vi "Alarm_CompareToThresholds.vi"(11 "HDF5_file_refs":T4 {"10HzRefs"."FileRef" format="%.0x"; "10HzRefs"."84Co_dset" format="%.0x"; "10HzRefs"."72Co_dset" format="%.0x"; "AlarmCfg"."84X_CalTonePwr"."ErrsAndWarns" scale=-120.0..-45.0; "AlarmCfg"."72X_CalTonePwr"."ErrsAndWarns" scale=-120.0..-45.0; "AlarmCfg"."84Co_CalTonePwr"."ErrsAndWarns" scale=-120.0..-45.0; "AlarmCfg"."72Co_CalTonePwr"."ErrsAndWarns" scale=-120.0..-45.0; "AlarmCfg"."84CoCalFreq"."ErrsAndWarns" scale=24.9..25.1; "AlarmCfg"."84CoBeacFreq"."ErrsAndWarns" scale=25.5..27.0; "AlarmCfg"."72CoCalFreq"."ErrsAndWarns" scale=24.9..25.1; "AlarmCfg"."72CoBeacFreq"."ErrsAndWarns" scale=25.5..27.0; "AlarmCfg"."ADAM4"."ErrsAndWarns" scale=30.0..52.0; "AlarmCfg"."ADAM3"."ErrsAndWarns" scale=30.0..52.0; "AlarmCfg"."ADAM2"."ErrsAndWarns" scale=30.0..52.0; "AlarmCfg"."ADAM1"."ErrsAndWarns" scale=30.0..52.0; "AlarmCfg"."TE3"."ErrsAndWarns" scale=30.0..52.0; "AlarmCfg"."TE2"."ErrsAndWarns" scale=30.0..52.0; "AlarmCfg"."TE1"."ErrsAndWarns" scale=20.0..52.0; "AlarmCfg"."AI19"."ErrsAndWarns" scale=0.0..60.0; "AlarmCfg"."AI18"."ErrsAndWarns" scale=-10.0..10.0; "AlarmCfg"."AI6"."ErrsAndWarns" scale=0.0..35.0; "AlarmCfg"."AI5"."ErrsAndWarns" scale=0.0..20.0; "AlarmCfg"."AI4"."ErrsAndWarns" scale=0.0..15.0; "AlarmCfg"."AI3"."ErrsAndWarns" scale=0.0..10.0; "AlarmCfg"."AI2"."ErrsAndWarns" scale=0.0..10.0; "AlarmCfg"."TC13"."ErrsAndWarns" scale=-10.0..40.0; "LogData"."NoiseInfo"."HDF5_NoiseInfo"."Sum" format="%^#.1g"; "HDFRefs2"."Complex"."Group_ref" format="%.0x"; "HDFRefs2"."Complex"."QSpect_dset" format="%.0x"; "HDFRefs2"."Complex"."ISpect_dset" format="%.0x"; "HDFRefs2"."Complex"."PwrSpect_dset" format="%.0x"; "HDFRefs2"."Complex"."TImeStamp_dset" format="%.0x"; "HDFRefs2"."ADAM_Refs"."Group_ref" format="%.0x"; "HDFRefs2"."ADAM_Refs"."ADAM_CoPol_dset" format="%.0x"; "HDFRefs2"."ADAM_Refs"."ADAM_XPol_dset" format="%.0x"; "HDFRefs2"."ADAM_Refs"."ADAM_Noise_dset" format="%.0x"; "HDFRefs2"."ADAM_Refs"."ADAM_CalBox_dset" format="%.0x"; "HDFRefs2"."ADAM_Refs"."TimeStamp" format="%.0x"; "HDFRefs2"."Filter_Refs"."Filter_Group_ref" format="%.0x"; "HDFRefs2"."Filter_Refs"."TimeStamp_dset" format="%.0x"; "HDFRefs2"."Filter_Refs"."Filter_dset" format="%.0x"; "HDFRefs2"."AI_Refs"."BlowerPwr_dset" format="%.0x"; "HDFRefs2"."AI_Refs"."ElStdDev_dset" format="%.0x"; "HDFRefs2"."AI_Refs"."AzStdDev_dset" format="%.0x"; "HDFRefs2"."AI_Refs"."AI19_dset" format="%.0x"; "HDFRefs2"."AI_Refs"."AI18_dset" format="%.0x"; "HDFRefs2"."AI_Refs"."AI17_dset" format="%.0x"; "HDFRefs2"."AI_Refs"."AI16_dset" format="%.0x"; "HDFRefs2"."AI_Refs"."AI6_dset" format="%.0x"; "HDFRefs2"."AI_Refs"."AI5_dset" format="%.0x"; "HDFRefs2"."AI_Refs"."AI4_dset" format="%.0x"; "HDFRefs2"."AI_Refs"."AI3_dset" format="%.0x"; "HDFRefs2"."AI_Refs"."AI2_dset" format="%.0x"; "HDFRefs2"."AI_Refs"."AI0_dset" format="%.0x"; "HDFRefs2"."AI_Refs"."AI1_dset" format="%.0x"; "HDFRefs2"."AI_Refs"."TimeString_dset" format="%.0x"; "HDFRefs2"."AI_Refs"."TimeStamp_dset" format="%.0x"; "HDFRefs2"."AI_Refs"."Group_ref" format="%.0x"; "HDFRefs2"."Weath_Refs"."WindDirSTD_dset" format="%.0x"; "HDFRefs2"."Weath_Refs"."WindGusts_dset" format="%.0x"; "HDFRefs2"."Weath_Refs"."RainFall_dset" format="%.0x"; "HDFRefs2"."Weath_Refs"."RainRate_dset" format="%.0x"; "HDFRefs2"."Weath_Refs"."Pressure_dset" format="%.0x"; "HDFRefs2"."Weath_Refs"."Humidity_dset" format="%.0x"; "HDFRefs2"."Weath_Refs"."Temp_dset" format="%.0x"; "HDFRefs2"."Weath_Refs"."WindDir_dset" format="%.0x"; "HDFRefs2"."Weath_Refs"."WindSpd_dset" format="%.0x"; "HDFRefs2"."Weath_Refs"."TimeStamp_dset" format="%.0x"; "HDFRefs2"."Weath_Refs"."Group_ref" format="%.0x"; "HDFRefs2"."Weath_Refs"."TimeString_dset" format="%.0x"; "HDFRefs2"."UPS_Refs_Deprecated"."TimeStamp_dset" format="%.0x"; "HDFRefs2"."UPS_Refs_Deprecated"."TimeString_dset" format="%.0x"; "HDFRefs2"."UPS_Refs_Deprecated"."%_dset" format="%.0x"; "HDFRefs2"."UPS_Refs_Deprecated"."W_dset" format="%.0x"; "HDFRefs2"."UPS_Refs_Deprecated"."Hz_dset" format="%.0x"; "HDFRefs2"."UPS_Refs_Deprecated"."A_dset" format="%.0x"; "HDFRefs2"."UPS_Refs_Deprecated"."V_dset" format="%.0x"; "HDFRefs2"."UPS_Refs_Deprecated"."Group_ref" format="%.0x"; "HDFRefs2"."TE_Refs"."TimeStamp" format="%.0x"; "HDFRefs2"."TE_Refs"."TE_Outp3_dset" format="%.0x"; "HDFRefs2"."TE_Refs"."TE_Temp3_dset" format="%.0x"; "HDFRefs2"."TE_Refs"."TE_Outp2_dset" format="%.0x"; "HDFRefs2"."TE_Refs"."TE_Temp2_dset" format="%.0x"; "HDFRefs2"."TE_Refs"."TE_Outp1_dset" format="%.0x"; "HDFRefs2"."TE_Refs"."TE_Temp1_dset" format="%.0x"; "HDFRefs2"."TE_Refs"."Group_ref" format="%.0x"; "HDFRefs2"."DisdromRefs"."Status_dset_deprecated" format="%.0x"; "HDFRefs2"."DisdromRefs"."Spectrum_dset" format="%.0x"; "HDFRefs2"."DisdromRefs"."SpectGroup_ref" format="%.0x"; "HDFRefs2"."DisdromRefs"."HydromType_dset" format="%.0x"; "HDFRefs2"."DisdromRefs"."UnknownVolum_dset" format="%.0x"; "HDFRefs2"."DisdromRefs"."UnknownParticls_dset" format="%.0x"; "HDFRefs2"."DisdromRefs"."NonHydrVolum_dset" format="%.0x"; "HDFRefs2"."DisdromRefs"."NonHydrParticls_dset" format="%.0x"; "HDFRefs2"."DisdromRefs"."ParticlMinDiam_dset" format="%.0x"; "HDFRefs2"."DisdromRefs"."ParticlMaxSpeed_dset" format="%.0x"; "HDFRefs2"."DisdromRefs"."RadarReflect_dset" format="%.0x"; "HDFRefs2"."DisdromRefs"."Visibility_dset" format="%.0x"; "HDFRefs2"."DisdromRefs"."TotalRain_dset" format="%.0x"; "HDFRefs2"."DisdromRefs"."Solid_dset" format="%.0x"; "HDFRefs2"."DisdromRefs"."Liquid_dset" format="%.0x"; "HDFRefs2"."DisdromRefs"."TotalRainRate_dset" format="%.0x"; "HDFRefs2"."DisdromRefs"."TimeStamp_dset" format="%.0x"; "HDFRefs2"."DisdromRefs"."ParticlMinSpeed_dset" format="%.0x"; "HDFRefs2"."DisdromRefs"."MeasdParticles_dset" format="%.0x"; "HDFRefs2"."DisdromRefs"."MaxDiam_dset" format="%.0x"; "HDFRefs2"."DisdromRefs"."BasicGroup_ref" format="%.0x"; "HDFRefs2"."ValidRefs"."Alarm_Source_dset" format="%.0x"; "HDFRefs2"."ValidRefs"."Time_AlarmChange_dset" format="%.0x"; "HDFRefs2"."ValidRefs"."Time_Valid_dset" format="%.0x"; "HDFRefs2"."ValidRefs"."Alarm_Valid_dset" format="%.0x"; "HDFRefs2"."ValidRefs"."Saturat_dset" format="%.0x"; "HDFRefs2"."ValidRefs"."Group_ref" format="%.0x"; "HDFRefs2"."ValidRefs"."Weath_Valid_dset" format="%.0x"; "HDFRefs2"."ValidRefs"."Disdr_Valid_dset" format="%.0x"; "HDFRefs2"."TC_Refs"."TC13_Tamb_Inter" format="%.0x"; "HDFRefs2"."TC_Refs"."TC12_Gen_Exhaust" format="%.0x"; "HDFRefs2"."TC_Refs"."TC11_HVAC_Cond_Out" format="%.0x"; "HDFRefs2"."TC_Refs"."TC10_HVAC_Cond_In" format="%.0x"; "HDFRefs2"."TC_Refs"."TC9_LP2_Lo" format="%.0x"; "HDFRefs2"."TC_Refs"."TC8_LP2_LoMid" format="%.0x"; "HDFRefs2"."TC_Refs"."TC7_LP2_Mid" format="%.0x"; "HDFRefs2"."TC_Refs"."TC6_LP2_MidHi" format="%.0x"; "HDFRefs2"."TC_Refs"."TC5_LP2_Hi" format="%.0x"; "HDFRefs2"."TC_Refs"."TC4_LP1_Lo" format="%.0x"; "HDFRefs2"."TC_Refs"."TC3_LP1_LoMid" format="%.0x"; "HDFRefs2"."TC_Refs"."TC2_LP1_Mid" format="%.0x"; "HDFRefs2"."TC_Refs"."TC1_LP1_MidHi" format="%.0x"; "HDFRefs2"."TC_Refs"."TC0_LP1_Hi" format="%.0x"; "HDFRefs2"."TC_Refs"."TimeString_dset" format="%.0x"; "HDFRefs2"."TC_Refs"."TimeStamp_dset" format="%.0x"; "HDFRefs2"."TC_Refs"."Group_ref" format="%.0x"; "HDFRefs2"."NoiseRefs"."TimeStamp_df_dset" format="%.0x"; "HDFRefs2"."NoiseRefs"."sum_dset" format="%.0x"; "HDFRefs2"."NoiseRefs"."df_dset" format="%.0x"; "HDFRefs2"."NoiseRefs"."TimeStamp_dset" format="%.0x"; "HDFRefs2"."NoiseRefs"."SumdSpectrum_dset" format="%.0x"; "HDFRefs2"."NoiseRefs"."TimeString_dset" format="%.0x"; "HDFRefs2"."NoiseRefs"."Group_ref" format="%.0x"; "HDFRefs2"."ToneRefs"."Group_ref" format="%.0x"; "HDFRefs2"."ToneRefs"."Cal"."Downshift_dset" format="%.0x"; "HDFRefs2"."ToneRefs"."Cal"."DeltaPhase_dset" format="%.0x"; "HDFRefs2"."ToneRefs"."Cal"."Phase_dset" format="%.0x"; "HDFRefs2"."ToneRefs"."Cal"."SNR_dset" format="%.0x"; "HDFRefs2"."ToneRefs"."Cal"."df_dset" format="%.0x"; "HDFRefs2"."ToneRefs"."Cal"."PeakLoc_dset" format="%.0x"; "HDFRefs2"."ToneRefs"."Cal"."MaxValue_dset" format="%.0x"; "HDFRefs2"."ToneRefs"."Cal"."TImeStamp_dset" format="%.0x"; "HDFRefs2"."ToneRefs"."Cal"."TimeString_dset" format="%.0x"; "HDFRefs2"."ToneRefs"."Beac"."Downshift_dset" format="%.0x"; "HDFRefs2"."ToneRefs"."Beac"."DeltaPhase_dset" format="%.0x"; "HDFRefs2"."ToneRefs"."Beac"."Phase_dset" format="%.0x"; "HDFRefs2"."ToneRefs"."Beac"."SNR_dset" format="%.0x"; "HDFRefs2"."ToneRefs"."Beac"."df_dset" format="%.0x"; "HDFRefs2"."ToneRefs"."Beac"."PeakLoc_dset" format="%.0x"; "HDFRefs2"."ToneRefs"."Beac"."MaxValue_dset" format="%.0x"; "HDFRefs2"."ToneRefs"."Beac"."TImeStamp_dset" format="%.0x"; "HDFRefs2"."ToneRefs"."Beac"."TimeString_dset" format="%.0x"; "HDFRefs2"."ToneRefs"."CalZoom_dSet" format="%.0x"; "HDFRefs2"."ToneRefs"."BeacZoom_dSet" format="%.0x"; "HDFRefs2"."File" format="%.0x"; "HDFRefs1"."Complex"."Group_ref" format="%.0x"; "HDFRefs1"."Complex"."QSpect_dset" format="%.0x"; "HDFRefs1"."Complex"."ISpect_dset" format="%.0x"; "HDFRefs1"."Complex"."PwrSpect_dset" format="%.0x"; "HDFRefs1"."Complex"."TImeStamp_dset" format="%.0x"; "HDFRefs1"."ADAM_Refs"."Group_ref" format="%.0x"; "HDFRefs1"."ADAM_Refs"."ADAM_CoPol_dset" format="%.0x"; "HDFRefs1"."ADAM_Refs"."ADAM_XPol_dset" format="%.0x"; "HDFRefs1"."ADAM_Refs"."ADAM_Noise_dset" format="%.0x"; "HDFRefs1"."ADAM_Refs"."ADAM_CalBox_dset" format="%.0x"; "HDFRefs1"."ADAM_Refs"."TimeStamp" format="%.0x"; "HDFRefs1"."Filter_Refs"."Filter_Group_ref" format="%.0x"; "HDFRefs1"."Filter_Refs"."TimeStamp_dset" format="%.0x"; "HDFRefs1"."Filter_Refs"."Filter_dset" format="%.0x"; "HDFRefs1"."AI_Refs"."BlowerPwr_dset" format="%.0x"; "HDFRefs1"."AI_Refs"."ElStdDev_dset" format="%.0x"; "HDFRefs1"."AI_Refs"."AzStdDev_dset" format="%.0x"; "HDFRefs1"."AI_Refs"."AI19_dset" format="%.0x"; "HDFRefs1"."AI_Refs"."AI18_dset" format="%.0x"; "HDFRefs1"."AI_Refs"."AI17_dset" format="%.0x"; "HDFRefs1"."AI_Refs"."AI16_dset" format="%.0x"; "HDFRefs1"."AI_Refs"."AI6_dset" format="%.0x"; "HDFRefs1"."AI_Refs"."AI5_dset" format="%.0x"; "HDFRefs1"."AI_Refs"."AI4_dset" format="%.0x"; "HDFRefs1"."AI_Refs"."AI3_dset" format="%.0x"; "HDFRefs1"."AI_Refs"."AI2_dset" format="%.0x"; "HDFRefs1"."AI_Refs"."AI0_dset" format="%.0x"; "HDFRefs1"."AI_Refs"."AI1_dset" format="%.0x"; "HDFRefs1"."AI_Refs"."TimeString_dset" format="%.0x"; "HDFRefs1"."AI_Refs"."TimeStamp_dset" format="%.0x"; "HDFRefs1"."AI_Refs"."Group_ref" format="%.0x"; "HDFRefs1"."Weath_Refs"."WindDirSTD_dset" format="%.0x"; "HDFRefs1"."Weath_Refs"."WindGusts_dset" format="%.0x"; "HDFRefs1"."Weath_Refs"."RainFall_dset" format="%.0x"; "HDFRefs1"."Weath_Refs"."RainRate_dset" format="%.0x"; "HDFRefs1"."Weath_Refs"."Pressure_dset" format="%.0x"; "HDFRefs1"."Weath_Refs"."Humidity_dset" format="%.0x"; "HDFRefs1"."Weath_Refs"."Temp_dset" format="%.0x"; "HDFRefs1"."Weath_Refs"."WindDir_dset" format="%.0x"; "HDFRefs1"."Weath_Refs"."WindSpd_dset" format="%.0x"; "HDFRefs1"."Weath_Refs"."TimeStamp_dset" format="%.0x"; "HDFRefs1"."Weath_Refs"."Group_ref" format="%.0x"; "HDFRefs1"."Weath_Refs"."TimeString_dset" format="%.0x"; "HDFRefs1"."UPS_Refs_Deprecated"."TimeStamp_dset" format="%.0x"; "HDFRefs1"."UPS_Refs_Deprecated"."TimeString_dset" format="%.0x"; "HDFRefs1"."UPS_Refs_Deprecated"."%_dset" format="%.0x"; "HDFRefs1"."UPS_Refs_Deprecated"."W_dset" format="%.0x"; "HDFRefs1"."UPS_Refs_Deprecated"."Hz_dset" format="%.0x"; "HDFRefs1"."UPS_Refs_Deprecated"."A_dset" format="%.0x"; "HDFRefs1"."UPS_Refs_Deprecated"."V_dset" format="%.0x"; "HDFRefs1"."UPS_Refs_Deprecated"."Group_ref" format="%.0x"; "HDFRefs1"."TE_Refs"."TimeStamp" format="%.0x"; "HDFRefs1"."TE_Refs"."TE_Outp3_dset" format="%.0x"; "HDFRefs1"."TE_Refs"."TE_Temp3_dset" format="%.0x"; "HDFRefs1"."TE_Refs"."TE_Outp2_dset" format="%.0x"; "HDFRefs1"."TE_Refs"."TE_Temp2_dset" format="%.0x"; "HDFRefs1"."TE_Refs"."TE_Outp1_dset" format="%.0x"; "HDFRefs1"."TE_Refs"."TE_Temp1_dset" format="%.0x"; "HDFRefs1"."TE_Refs"."Group_ref" format="%.0x"; "HDFRefs1"."DisdromRefs"."Status_dset_deprecated" format="%.0x"; "HDFRefs1"."DisdromRefs"."Spectrum_dset" format="%.0x"; "HDFRefs1"."DisdromRefs"."SpectGroup_ref" format="%.0x"; "HDFRefs1"."DisdromRefs"."HydromType_dset" format="%.0x"; "HDFRefs1"."DisdromRefs"."UnknownVolum_dset" format="%.0x"; "HDFRefs1"."DisdromRefs"."UnknownParticls_dset" format="%.0x"; "HDFRefs1"."DisdromRefs"."NonHydrVolum_dset" format="%.0x"; "HDFRefs1"."DisdromRefs"."NonHydrParticls_dset" format="%.0x"; "HDFRefs1"."DisdromRefs"."ParticlMinDiam_dset" format="%.0x"; "HDFRefs1"."DisdromRefs"."ParticlMaxSpeed_dset" format="%.0x"; "HDFRefs1"."DisdromRefs"."RadarReflect_dset" format="%.0x"; "HDFRefs1"."DisdromRefs"."Visibility_dset" format="%.0x"; "HDFRefs1"."DisdromRefs"."TotalRain_dset" format="%.0x"; "HDFRefs1"."DisdromRefs"."Solid_dset" format="%.0x"; "HDFRefs1"."DisdromRefs"."Liquid_dset" format="%.0x"; "HDFRefs1"."DisdromRefs"."TotalRainRate_dset" format="%.0x"; "HDFRefs1"."DisdromRefs"."TimeStamp_dset" format="%.0x"; "HDFRefs1"."DisdromRefs"."ParticlMinSpeed_dset" format="%.0x"; "HDFRefs1"."DisdromRefs"."MeasdParticles_dset" format="%.0x"; "HDFRefs1"."DisdromRefs"."MaxDiam_dset" format="%.0x"; "HDFRefs1"."DisdromRefs"."BasicGroup_ref" format="%.0x"; "HDFRefs1"."ValidRefs"."Alarm_Source_dset" format="%.0x"; "HDFRefs1"."ValidRefs"."Time_AlarmChange_dset" format="%.0x"; "HDFRefs1"."ValidRefs"."Time_Valid_dset" format="%.0x"; "HDFRefs1"."ValidRefs"."Alarm_Valid_dset" format="%.0x"; "HDFRefs1"."ValidRefs"."Saturat_dset" format="%.0x"; "HDFRefs1"."ValidRefs"."Group_ref" format="%.0x"; "HDFRefs1"."ValidRefs"."Weath_Valid_dset" format="%.0x"; "HDFRefs1"."ValidRefs"."Disdr_Valid_dset" format="%.0x"; "HDFRefs1"."TC_Refs"."TC13_Tamb_Inter" format="%.0x"; "HDFRefs1"."TC_Refs"."TC12_Gen_Exhaust" format="%.0x"; "HDFRefs1"."TC_Refs"."TC11_HVAC_Cond_Out" format="%.0x"; "HDFRefs1"."TC_Refs"."TC10_HVAC_Cond_In" format="%.0x"; "HDFRefs1"."TC_Refs"."TC9_LP2_Lo" format="%.0x"; "HDFRefs1"."TC_Refs"."TC8_LP2_LoMid" format="%.0x"; "HDFRefs1"."TC_Refs"."TC7_LP2_Mid" format="%.0x"; "HDFRefs1"."TC_Refs"."TC6_LP2_MidHi" format="%.0x"; "HDFRefs1"."TC_Refs"."TC5_LP2_Hi" format="%.0x"; "HDFRefs1"."TC_Refs"."TC4_LP1_Lo" format="%.0x"; "HDFRefs1"."TC_Refs"."TC3_LP1_LoMid" format="%.0x"; "HDFRefs1"."TC_Refs"."TC2_LP1_Mid" format="%.0x"; "HDFRefs1"."TC_Refs"."TC1_LP1_MidHi" format="%.0x"; "HDFRefs1"."TC_Refs"."TC0_LP1_Hi" format="%.0x"; "HDFRefs1"."TC_Refs"."TimeString_dset" format="%.0x"; "HDFRefs1"."TC_Refs"."TimeStamp_dset" format="%.0x"; "HDFRefs1"."TC_Refs"."Group_ref" format="%.0x"; "HDFRefs1"."NoiseRefs"."TimeStamp_df_dset" format="%.0x"; "HDFRefs1"."NoiseRefs"."sum_dset" format="%.0x"; "HDFRefs1"."NoiseRefs"."df_dset" format="%.0x"; "HDFRefs1"."NoiseRefs"."TimeStamp_dset" format="%.0x"; "HDFRefs1"."NoiseRefs"."SumdSpectrum_dset" format="%.0x"; "HDFRefs1"."NoiseRefs"."TimeString_dset" format="%.0x"; "HDFRefs1"."NoiseRefs"."Group_ref" format="%.0x"; "HDFRefs1"."ToneRefs"."Group_ref" format="%.0x"; "HDFRefs1"."ToneRefs"."Cal"."Downshift_dset" format="%.0x"; "HDFRefs1"."ToneRefs"."Cal"."DeltaPhase_dset" format="%.0x"; "HDFRefs1"."ToneRefs"."Cal"."Phase_dset" format="%.0x"; "HDFRefs1"."ToneRefs"."Cal"."SNR_dset" format="%.0x"; "HDFRefs1"."ToneRefs"."Cal"."df_dset" format="%.0x"; "HDFRefs1"."ToneRefs"."Cal"."PeakLoc_dset" format="%.0x"; "HDFRefs1"."ToneRefs"."Cal"."MaxValue_dset" format="%.0x"; "HDFRefs1"."ToneRefs"."Cal"."TImeStamp_dset" format="%.0x"; "HDFRefs1"."ToneRefs"."Cal"."TimeString_dset" format="%.0x"; "HDFRefs1"."ToneRefs"."Beac"."Downshift_dset" format="%.0x"; "HDFRefs1"."ToneRefs"."Beac"."DeltaPhase_dset" format="%.0x"; "HDFRefs1"."ToneRefs"."Beac"."Phase_dset" format="%.0x"; "HDFRefs1"."ToneRefs"."Beac"."SNR_dset" format="%.0x"; "HDFRefs1"."ToneRefs"."Beac"."df_dset" format="%.0x"; "HDFRefs1"."ToneRefs"."Beac"."PeakLoc_dset" format="%.0x"; "HDFRefs1"."ToneRefs"."Beac"."MaxValue_dset" format="%.0x"; "HDFRefs1"."ToneRefs"."Beac"."TImeStamp_dset" format="%.0x"; "HDFRefs1"."ToneRefs"."Beac"."TimeString_dset" format="%.0x"; "HDFRefs1"."ToneRefs"."CalZoom_dSet" format="%.0x"; "HDFRefs1"."ToneRefs"."BeacZoom_dSet" format="%.0x"; "HDFRefs1"."File" format="%.0x"; "Config"."FP_User"."Deadband" format="%#.0f"}) -> (1 "AllAlarms":T2[](array[typedef]), 2 "Alarm Status":T3, 3 "WeatherStatus":bool[](array[boolean]), 4 "Elapsed_SNR_Timer":dbl, 5 "SaturationStatus":T1)   [LabVIEW 2018]
uses:
  Controls/Clusts/LogLoopClust.ctl
  Controls/Clusts/Config_Clust.ctl
  Controls/Clusts/UserConfig.ctl
  Controls/PathsCluster.ctl
  Controls/Clusts/FrontPanel_UserConfig.ctl
  Controls/Clusts/Inclinometer_User_Cfg.ctl
  Controls/Clusts/FP_UserTargetConfig.ctl
  Controls/Clusts/FreqShift.ctl
  Controls/Clusts/FPGA_Scale.ctl
  Controls/Enums/ScaleMeasure.ctl
  Controls/RadioButtons/FilterEnableRadio.ctl
  Controls/Enums/TargetNumber.ctl
  Controls/Clusts/HDF5_File_Refs.ctl
  <vilib>/addons/h5labview2/base/hid_t.ctl
  Controls/Clusts/ToneGroupRefsClust.ctl
  HDF5/HDF5_Tone_refs.ctl
  HDF5/HDF5_Noise_refs.ctl
  HDF5/TC_Tone_refs.ctl
  HDF5/HDF5_Validty_refs.ctl
  HDF5/HDF5_Disdrometer_Refs.ctl
  HDF5/HDF5_Health_Refs.ctl
  HDF5/UPS_refs.ctl
  Controls/Clusts/WeatherRefs.ctl
  HDF5/HDF5_AI_refs.ctl
  HDF5/HDF5_Filter_refs.ctl
  HDF5/HDF5_ADAM_Refs.ctl
  HDF5/HDF5_Complex_Refs.ctl
  Controls/Clusts/LogDataClust.ctl
  Controls/Clusts/ToneLogBuffered.ctl
  Controls/Clusts/SaturationMonitorBuffer.ctl
  HDF5/TC_Data_Structure.ctl
  Controls/Clusts/AI_Clust.ctl
  HDF5/HDF5_NoiseInfoClust.ctl
  HDF5/DisdrometerData.ctl
  HDF5/DisdromterSummaryData.ctl
  Disdrometer/Disdrometer_Status_Cluster.ctl
  Controls/Clusts/WeatherDataClust.ctl
  Controls/Clusts/ValidityWeatherClust.ctl
  Controls/Clusts/TE_Data_Clust.ctl
  HDF5/HDF5_ADAM_Data.ctl
  Controls/Clusts/TimeDomainData.ctl
  Controls/Clusts/AlarmSettingsClust.ctl
  Controls/Clusts/AlarmThresh_OneChan.ctl
  Controls/Clusts/ErrorStatus.ctl
  Controls/Clusts/DigOutClust.ctl
  Controls/Clusts/Saturation_Status_Clust.ctl
  Controls/Clusts/HDF5_10HzRefs.ctl
types:
  T1 = typedef "Saturation_Status_Clust.ctl" = cluster{"84":bool[], "72":bool[]}
  T2 = typedef "ErrorStatus.ctl" = cluster{"RX?":bool, "Warn":bool, "Error":bool, "Enabl":bool, "Source":string}
  T3 = typedef "DigOutClust.ctl" = cluster{"Green":bool, "Rx_Yell":bool, "Cx_Yell":bool, "Red":bool, "Source":string}
  T4 = typedef "LogLoopClust.ctl" = cluster{"base path":path, "PathNow1":path, "PathNow2":path, "DateNow":string, "NAS path":path, "LogFiltStage":bool, "LogNoise_df_1":bool, "LogNoise_df_2":bool, "LogNoise_df_3":bool, "LogNoise_df_4":bool, "Config":T5, "HDFRefs1":T16, "HDFRefs2":T16, "LogData":T31, "AlarmCfg":T45, "DO":bool[], "AllAlarms":T2[], "Alarm Status":T3, "SaturationStatus":T1, "WeatherStatus":bool[], "10HzRefs":T47}
  T5 = typedef "Config_Clust.ctl" = cluster{"UsrCfg":T6, "FP_User":T8}
  T6 = typedef "UserConfig.ctl" = cluster{"Paths":T7, "SampleRate":dbl}
  T7 = typedef "PathsCluster.ctl" = cluster{"CfgFile":path, "LogFolder":path, "LogFile":path, "NAS path":path, "ThreshFile":path, "RedunFolder":path}
  T8 = typedef "FrontPanel_UserConfig.ctl" = cluster{"#NoiseSums":u32, "Max_df":u32, "AvgAvg":bool, "#Avg":u16, "AutoCenter":bool, "Inclin":T9, "1":T10, "2":T10, "3":T10, "4":T10, "Target to Probe":T15, "SNR_Thresh":dbl, "Paths":T7, "Connex_Location":string, "SimulateFPGA":bool, "Deadband":dbl}
  T9 = typedef "Inclinometer_User_Cfg.ctl" = cluster{"Vmin":dbl, "Vmax":dbl, "Angle_min":dbl, "Angle_max":dbl, "Offset":dbl, "Pos_Neg":bool}
  T10 = typedef "FP_UserTargetConfig.ctl" = cluster{"Cal_":T11, "Beac":T11, "Scale":T12, "Offset":fxp<+/-,16,16>, "Scale_Noise":fxp<+/-,30,30>, "Scale_Step1":fxp<+/-,17,17>, "Scale_In_RT":ext, "ScaleMeas":fxp<+/-,16,1>, "FreqsToRemove":i32[], "Width":i32[], "ScaleMeasEnum":T13, "FilterEnab":T14}
  T11 = typedef "FreqShift.ctl" = cluster{"Fine":dbl, "Coarse_":dbl}
  T12 = typedef "FPGA_Scale.ctl" = cluster{"Step4":fxp<+/-,23,23>, "Step5":fxp<+/-,23,23>, "Step6":fxp<+/-,23,23>, "Step7":fxp<+/-,23,23>}
  T13 = typedef "ScaleMeasure.ctl" = enum16{"1", "10", "50", "42"}
  T14 = typedef "FilterEnableRadio.ctl" = enum32{"None", "Step 1", "Frequency Shift", "Step 4", "Step 5", "Step 6", "Step 7"}
  T15 = typedef "TargetNumber.ctl" = enum16{"1", "2", "3", "4"}
  T16 = typedef "HDF5_File_Refs.ctl" = cluster{"File":T17, "ToneRefs":T18[], "NoiseRefs":T20[], "TC_Refs":T21, "ValidRefs":T22, "DisdromRefs":T23, "TE_Refs":T24, "UPS_Refs_Deprecated":T25, "Weath_Refs":T26, "AI_Refs":T27, "Filter_Refs":T28, "ADAM_Refs":T29, "Complex":T30[]}
  T17 = typedef "hid_t.ctl" = i32
  T18 = typedef "ToneGroupRefsClust.ctl" = cluster{"Group_ref":T17, "Cal":T19, "Beac":T19, "CalZoom_dSet":T17, "BeacZoom_dSet":T17}
  T19 = typedef "HDF5_Tone_refs.ctl" = cluster{"TimeString_dset":T17, "TImeStamp_dset":T17, "SNR_dset":T17, "MaxValue_dset":T17, "PeakLoc_dset":T17, "df_dset":T17, "Phase_dset":T17, "DeltaPhase_dset":T17, "Downshift_dset":T17}
  T20 = typedef "HDF5_Noise_refs.ctl" = cluster{"Group_ref":T17, "TimeString_dset":T17, "TimeStamp_dset":T17, "TimeStamp_df_dset":T17, "df_dset":T17, "sum_dset":T17, "SumdSpectrum_dset":T17}
  T21 = typedef "TC_Tone_refs.ctl" = cluster{"Group_ref":T17, "TimeString_dset":T17, "TimeStamp_dset":T17, "TC0_LP1_Hi":T17, "TC1_LP1_MidHi":T17, "TC2_LP1_Mid":T17, "TC3_LP1_LoMid":T17, "TC4_LP1_Lo":T17, "TC5_LP2_Hi":T17, "TC6_LP2_MidHi":T17, "TC7_LP2_Mid":T17, "TC8_LP2_LoMid":T17, "TC9_LP2_Lo":T17, "TC10_HVAC_Cond_In":T17, "TC11_HVAC_Cond_Out":T17, "TC12_Gen_Exhaust":T17, "TC13_Tamb_Inter":T17}
  T22 = typedef "HDF5_Validty_refs.ctl" = cluster{"Group_ref":T17, "Weath_Valid_dset":T17, "Disdr_Valid_dset":T17, "Saturat_dset":T17, "Alarm_Valid_dset":T17, "Time_Valid_dset":T17, "Time_AlarmChange_dset":T17, "Alarm_Source_dset":T17}
  T23 = typedef "HDF5_Disdrometer_Refs.ctl" = cluster{"BasicGroup_ref":T17, "TimeStamp_dset":T17, "TotalRainRate_dset":T17, "Liquid_dset":T17, "Solid_dset":T17, "TotalRain_dset":T17, "Visibility_dset":T17, "RadarReflect_dset":T17, "MaxDiam_dset":T17, "MeasdParticles_dset":T17, "ParticlMinSpeed_dset":T17, "ParticlMaxSpeed_dset":T17, "ParticlMinDiam_dset":T17, "NonHydrParticls_dset":T17, "NonHydrVolum_dset":T17, "UnknownParticls_dset":T17, "UnknownVolum_dset":T17, "HydromType_dset":T17, "SpectGroup_ref":T17, "Spectrum_dset":T17, "Status_dset_deprecated":T17}
  T24 = typedef "HDF5_Health_Refs.ctl" = cluster{"Group_ref":T17, "TE_Temp1_dset":T17, "TE_Outp1_dset":T17, "TE_Temp2_dset":T17, "TE_Outp2_dset":T17, "TE_Temp3_dset":T17, "TE_Outp3_dset":T17, "TimeStamp":T17}
  T25 = typedef "UPS_refs.ctl" = cluster{"Group_ref":T17, "TimeString_dset":T17, "TimeStamp_dset":T17, "V_dset":T17, "A_dset":T17, "Hz_dset":T17, "W_dset":T17, "%_dset":T17}
  T26 = typedef "WeatherRefs.ctl" = cluster{"Group_ref":T17, "TimeString_dset":T17, "TimeStamp_dset ":T17, "WindSpd_dset":T17, "WindGusts_dset":T17, "WindDir_dset":T17, "WindDirSTD_dset":T17, "Temp_dset":T17, "Humidity_dset":T17, "Pressure_dset":T17, "RainRate_dset":T17, "RainFall_dset":T17}
  T27 = typedef "HDF5_AI_refs.ctl" = cluster{"Group_ref":T17, "TimeString_dset":T17, "TimeStamp_dset":T17, "AI0_dset":T17, "AI1_dset":T17, "AI2_dset":T17, "AI3_dset":T17, "AI4_dset":T17, "AI5_dset":T17, "AI6_dset":T17, "AI16_dset":T17, "AI17_dset":T17, "AI18_dset":T17, "AzStdDev_dset":T17, "AI19_dset":T17, "ElStdDev_dset":T17, "BlowerPwr_dset":T17}
  T28 = typedef "HDF5_Filter_refs.ctl" = cluster{"Filter_Group_ref":T17, "TimeStamp_dset":T17, "Filter_dset":T17}
  T29 = typedef "HDF5_ADAM_Refs.ctl" = cluster{"Group_ref":T17, "ADAM_CoPol_dset":T17, "ADAM_XPol_dset":T17, "ADAM_Noise_dset":T17, "ADAM_CalBox_dset":T17, "TimeStamp":T17}
  T30 = typedef "HDF5_Complex_Refs.ctl" = cluster{"Group_ref":T17, "TImeStamp_dset":T17, "PwrSpect_dset":T17, "ISpect_dset":T17, "QSpect_dset":T17}
  T31 = typedef "LogDataClust.ctl" = cluster{"Tone":T32[], "TCData":T34, "AI":T35, "NoiseTrace":cluster{"Target":T15, "NoiseTrace":dbl[]}[], "NoiseInfo":cluster{"Target":T15, "HDF5_NoiseInfo":T36}[], "Disdrom":T37[], "Weath":T40[], "TE":T42, "ADAM":T43, "TimeDomain":T44[]}
  T32 = typedef "ToneLogBuffered.ctl" = cluster{"Count":i32, "CalVal":sgl[], "CalLoc":i32[], "BeacVal":sgl[], "BeacLoc":i32[], "BeacShift":i32[], "Enum":T15, "df":dbl, "PwrSpectr":sgl[][], "ISpectr":sgl[][], "QSpectr":sgl[][], "Time":timestamp[], "SNR":sgl[], "AboveThresh":bool[], "10Hz_PeakVal":dbl[], "Phase":sgl[], "DeltaPhase":dbl[], "Saturat":T33, "10MHz":bool}
  T33 = typedef "SaturationMonitorBuffer.ctl" = cluster{"Meas":bool[], "Stage1":bool[], "Stage4":bool[], "Stage5":bool[], "Stage6":bool[], "Stage7":bool[]}
  T34 = typedef "TC_Data_Structure.ctl" = cluster{"TimeStamp":dbl, "TimeString":string, "TC0_LP1_Hi":dbl, "TC1_LP1_MidHi":dbl, "TC2_LP1_Mid":dbl, "TC3_LP1_LoMid":dbl, "TC4_LP1_Lo":dbl, "TC5_LP2_Hi":dbl, "TC6_LP2_MidHi":dbl, "TC7_LP2_Mid":dbl, "TC8_LP2_LoMid":dbl, "TC9_LP2_Lo":dbl, "TC10_HVAC_Cond_In":dbl, "TC11_HVAC_Cond_Out":dbl, "TC12_Gen_Exhaust":dbl, "TC13_Amb_Inter":dbl, "TC14_Unused":dbl, "TC15_Unused":dbl, "TC16_Unused":dbl, "TC17_Unused":dbl, "TC18_Unused":dbl, "TC19_Unused":dbl, "TC20_Unused":dbl, "TC21_Unused":dbl, "TC22_Unused":dbl, "TC23_Unused":dbl, "TC24_Unused":dbl, "TC25_Unused":dbl, "TC26_Unused":dbl, "TC27_Unused":dbl, "TC28_Unused":dbl, "TC29_Unused":dbl, "TC30_Unused":dbl, "TC31_Unused":dbl}
  T35 = typedef "AI_Clust.ctl" = cluster{"TimeString":string, "Time Stamp":dbl, "AI0_Unused":dbl, "AI1_-5V":dbl, "AI2_+5V":dbl, "AI3_+6V":dbl, "AI4_+12V":dbl, "AI5_+15V":dbl, "AI6_+28V":dbl, "AI7_Unused":dbl, "Ai16_72GHz_CalPower":dbl, "Ai17_84GHz_CalPower":dbl, "Ai18_InclinAz":dbl, "Ai19_InclinEl":dbl, "Ai20_BlowerPwr":dbl, "Ai21_Unused":dbl, "Ai22_Unused":dbl, "Ai23_Unused":dbl, "InclinA_StdDev":dbl, "InclinB_StdDev":dbl, "InclinAz_Unfilt":dbl, "InclinEl_Unfilt":dbl}
  T36 = typedef "HDF5_NoiseInfoClust.ctl" = cluster{"Timestring":string, "Timestamp":dbl, "df":dbl, "Sum":dbl}
  T37 = typedef "DisdrometerData.ctl" = cluster{"Spectrum Data":i16[], "DisdromSummary":T38, "Status":T39}
  T38 = typedef "DisdromterSummaryData.ctl" = cluster{"current time":dbl, "Timestamp":dbl, "Total Rain Rate":dbl, "Liquid Rain Rate":dbl, "Solid Rain Rate":dbl, "Total Rainfall":dbl, "Visibility":dbl, "Radar Reflectivity":dbl, "Max Diameter Hail":dbl, "Measured Particles":i32, "Particle Min Speed":i16, "Particle Max Speed":i16, "Particle Min Diam":i16, "NonHydr Particles":i16, "NonHydr Volume":dbl, "Unkn Particles":i16, "Unkn Volume":dbl, "HydroType":i8}
  T39 = typedef "Disdrometer_Status_Cluster.ctl" = cluster{"Laser":bool, "Signal":bool, "LaserTemp_Analog":bool, "LaserTemp_Digital":bool, "LaserCurrent_Analog":bool, "LaserCurrent_Digital":bool, "SensorSupply":bool, "HeatLaserHead":bool, "HeatReceiverHead":bool, "TempSensor":bool, "HeatSupply":bool, "HeatHousing":bool, "HeatHeads":bool, "HeatCarriers":bool, "OutputLaserPower":bool, "Checksum":bool, "StatusInt":u16}
  T40 = typedef "WeatherDataClust.ctl" = cluster{"TimeString":string, "Timestamp":dbl, "Wind Speed":sgl, "Wind Gusts":sgl, "Wind Dir":sgl, "Wind Dir STD":sgl, "Temperature":sgl, "Humidity":sgl, "Pressure":sgl, "Rain Rate":i16, "Rain Fall":sgl, "Status":T41}
  T41 = typedef "ValidityWeatherClust.ctl" = cluster{"Temp_OutOfBounds":bool, "Temp_IncrSTD":bool, "Temp_Oth":bool, "BarPress_OutOfBounds":bool, "BarPress_IncrSTD":bool, "BarPress_Change":bool, "BarPress_Other":bool, "Humid_OutOfBounds":bool, "Humid_IncrSTD":bool, "Humid_Other":bool, "Wind__Spd_OutOfBounds":bool, "Wind_Dir_OutOfBounds":bool, "RainBuck_OutOfBounds":bool, "RainBuck_Disdrom":bool, "Disdrom_RainBuck":bool, "Placeholder":bool}
  T42 = typedef "TE_Data_Clust.ctl" = cluster{"TimeString":string, "TimeStamp":dbl, "Temp":dbl, "Output":dbl, "Temp 2":dbl, "Output 2":dbl, "Temp 3":dbl, "Output 3":dbl}
  T43 = typedef "HDF5_ADAM_Data.ctl" = cluster{"Timestamp":dbl, "Time string":string, "Fault 1":bool, "Fault 2":bool, "Fault 3":bool, "Fault 4":bool, "Fault 5":bool, "Fault 6":bool, "Value 1":dbl, "Value 2":dbl, "Value 3":dbl, "Value 4":dbl, "Value 5":dbl, "Value 6":dbl}
  T44 = typedef "TimeDomainData.ctl" = cluster{"CalTimeVal":dbl[], "CalTimeCount":u32[], "Enum":T15}
  T45 = typedef "AlarmSettingsClust.ctl" = cluster{"TC13":T46, "AI1":T46, "AI2":T46, "AI3":T46, "AI4":T46, "AI5":T46, "AI6":T46, "AI18":T46, "AI19":T46, "TE1":T46, "TE2":T46, "TE3":T46, "ADAM1":T46, "ADAM2":T46, "ADAM3":T46, "ADAM4":T46, "72CoBeacFreq":T46, "72CoCalFreq":T46, "84CoBeacFreq":T46, "84CoCalFreq":T46, "72Co_CalTonePwr":T46, "72X_CalTonePwr":T46, "84Co_CalTonePwr":T46, "84X_CalTonePwr":T46}
  T46 = typedef "AlarmThresh_OneChan.ctl" = cluster{"Enbl":bool, "ErrsAndWarns":cluster{dbl, dbl, dbl, dbl}}
  T47 = typedef "HDF5_10HzRefs.ctl" = cluster{"72Co_dset":T17, "84Co_dset":T17, "FileRef":T17}
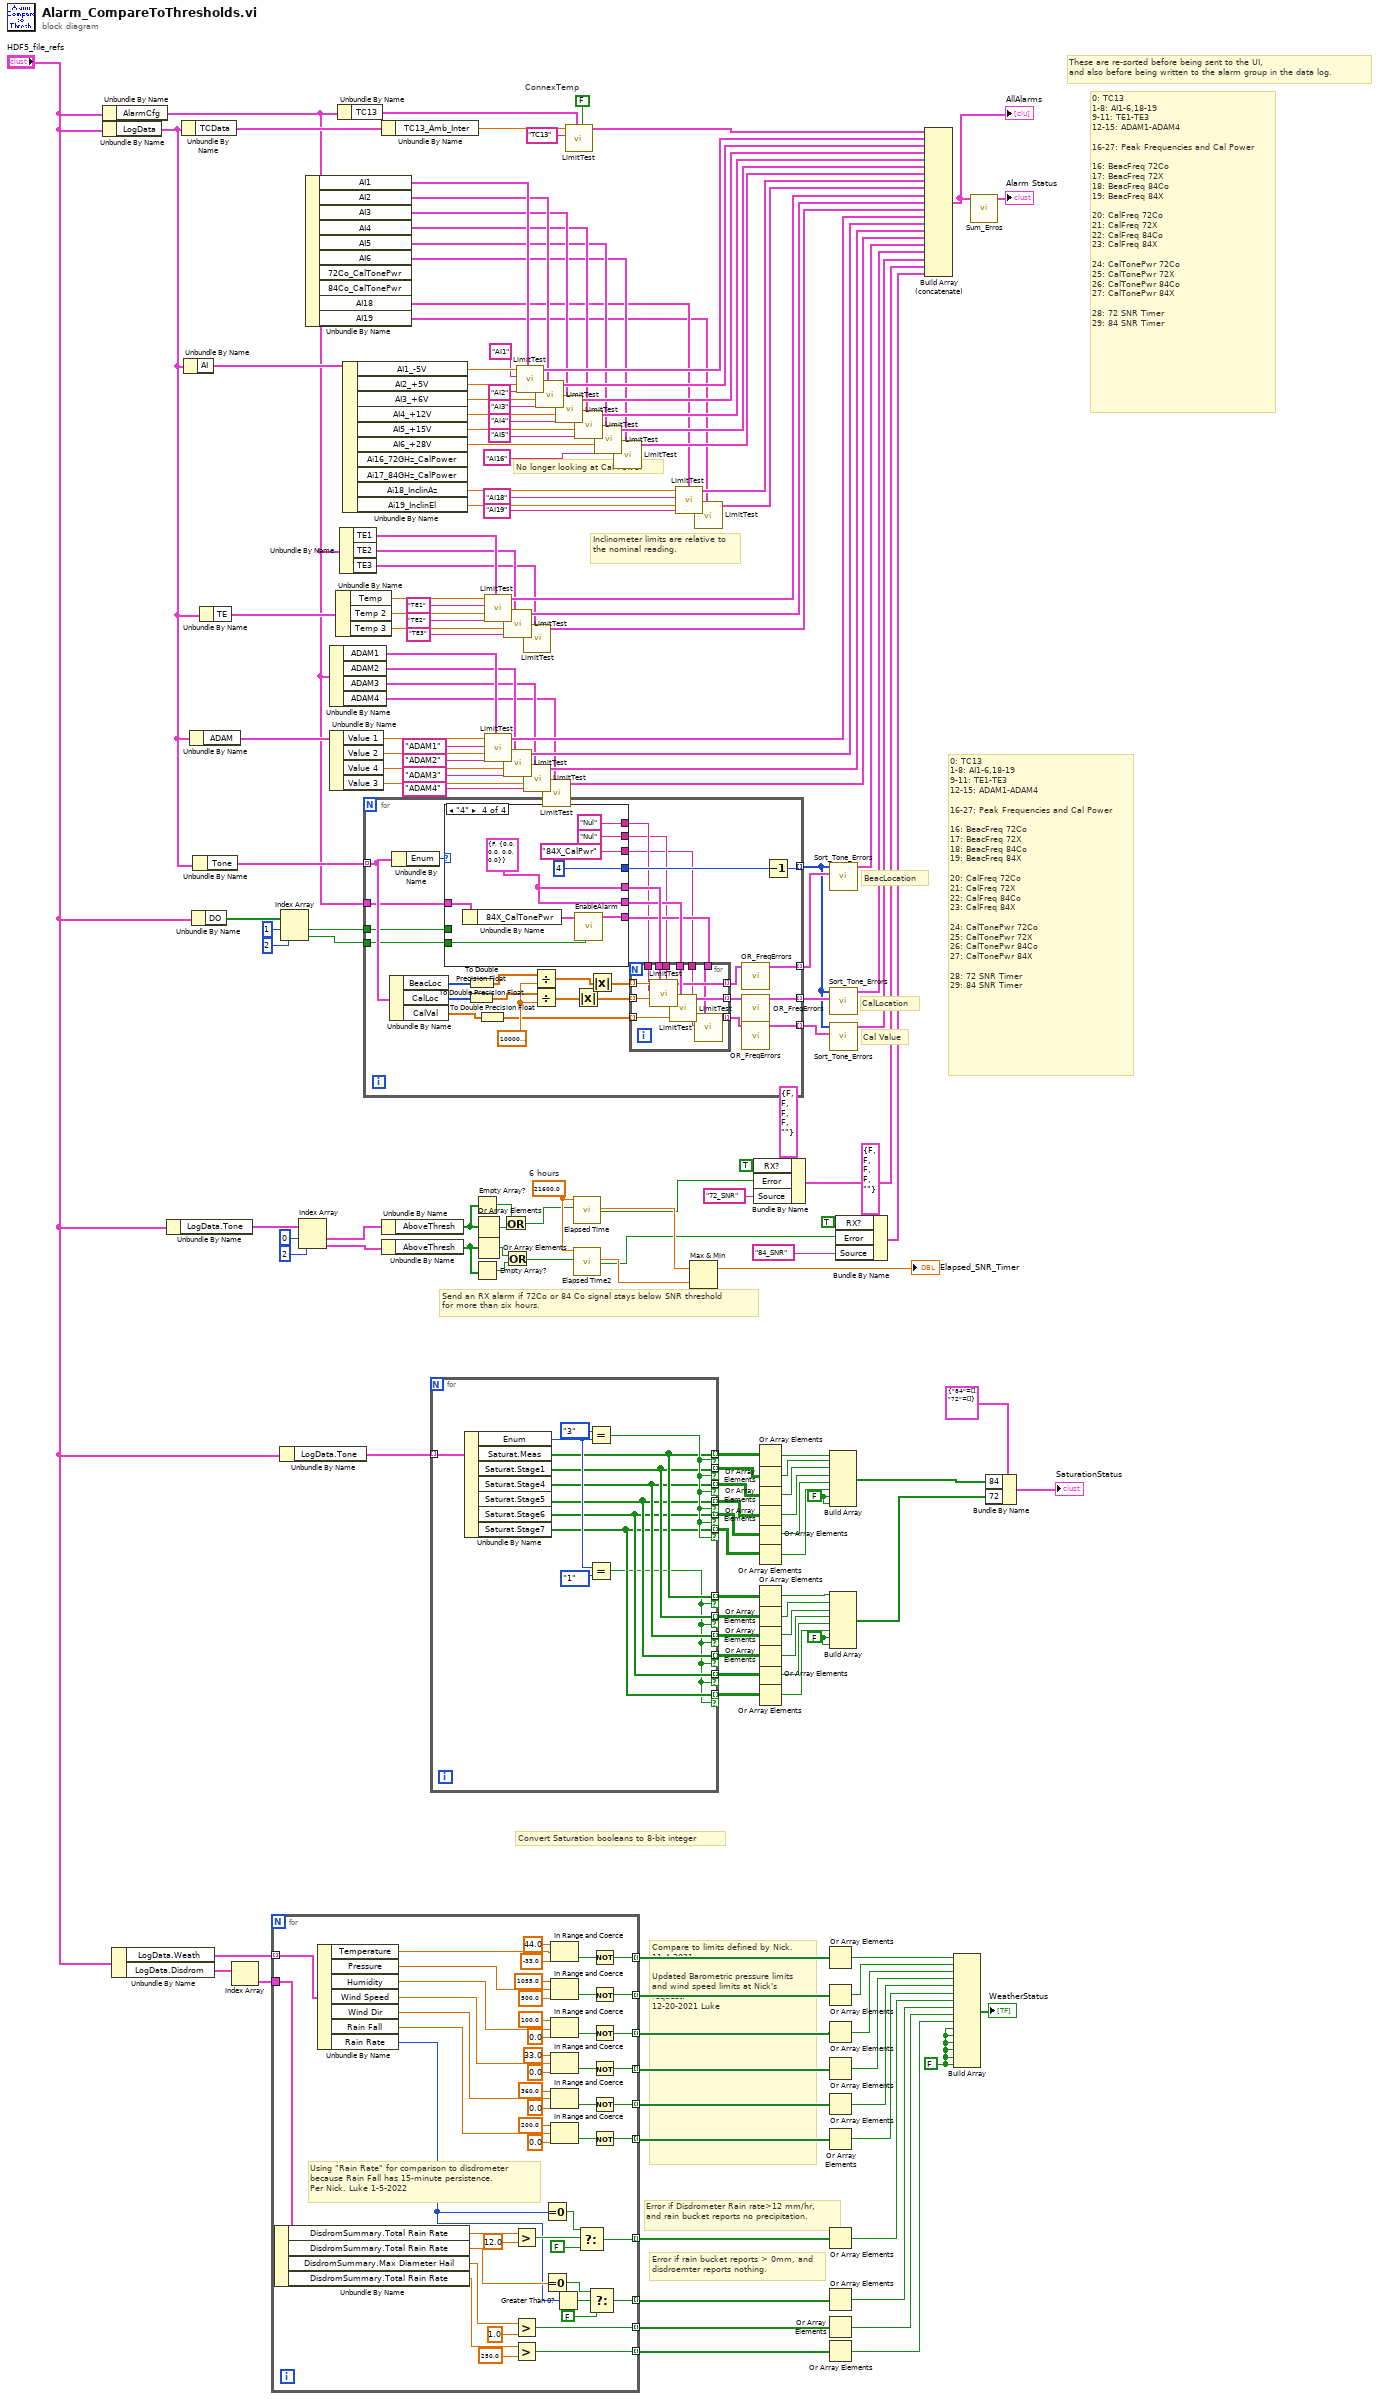
[diagram p0: block diagram]
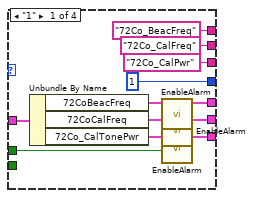
[diagram p2: hidden frame]
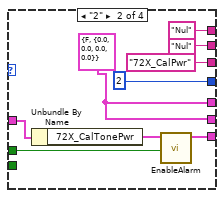
[diagram p3: hidden frame]
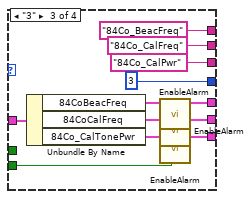
[diagram p4: hidden frame]
diagram:
  w20 = FALSE
  w66 = FALSE ("element")
  w74 = FALSE ("element")
  w94 = 21600.0  # 6 hours
  w125 = FALSE  # ConnexTemp
  # "Error if rain bucket reports > 0mm, and disdroemter reports nothing."
  # "Error if Disdrometer Rain rate>12 mm/hr, and rain bucket reports no precipitation."
  # "Compare to limits defined by Nick.\n11-4-2021\n\nUpdated Barometric pressure limits and wind speed limits at Nick's request.\n12-20-2021 Luke"
  # "0: TC13\n1-8: AI1-6,18-19\n9-11: TE1-TE3\n12-15: ADAM1-ADAM4\n\n16-27: Peak Frequencies and Cal Power\n\n16: BeacFreq 72Co \n17: BeacFreq 72X \n18: BeacFreq 84Co \n19: BeacFreq 84X\n \n20: CalFreq 72Co\n21: CalFreq 72X\n22: CalFreq 84Co\n23: CalFreq 84X\n \n24: CalTonePwr 72Co\n25: CalTonePwr 72X\n26: CalTonePwr 84Co\n27: CalTonePwr 84X\n\n28: 72 SNR Timer\n29: 84 SNR Timer"
  # "These are re-sorted before being sent to the UI,\nand also before being written to the alarm group in the data log."
  # "Cal Value"
  # "CalLocation"
  # "BeacLocation"
  # "Convert Saturation booleans to 8-bit integer"
  # "Send an RX alarm if 72Co or 84 Co signal stays below SNR threshold\nfor more than six hours."
  # "0: TC13\n1-8: AI1-6,18-19\n9-11: TE1-TE3\n12-15: ADAM1-ADAM4\n\n16-27: Peak Frequencies and Cal Power\n\n16: BeacFreq 72Co \n17: BeacFreq 72X \n18: BeacFreq 84Co \n19: BeacFreq 84X\n \n20: CalFreq 72Co\n21: CalFreq 72X\n22: CalFreq 84Co\n23: CalFreq 84X\n \n24: CalTonePwr 72Co\n25: CalTonePwr 72X\n26: CalTonePwr 84Co\n27: CalTonePwr 84X\n\n28: 72 SNR Timer\n29: 84 SNR Timer"
  # "No longer looking at Cal Power"
  # "Inclinometer limits are relative to the nominal reading."
  n1 = Unbundle By Name("HDF5_file_refs") -> ("AlarmCfg"=w151:T45)
  n2 = Unbundle By Name("HDF5_file_refs") -> ("LogData"=w110:T31)
  n3 = Unbundle By Name("HDF5_file_refs") -> ("LogData.Weath"=w43:T40[], "LogData.Disdrom"=w42:T37[])
  n4 = Unbundle By Name("HDF5_file_refs") -> ("LogData.Tone"=w101:T32[])
  n5 = Unbundle By Name(w110) -> ("TCData"=w168:T34)
  n6 = Unbundle By Name(w110) -> ("AI"=w170:T35)
  n7 = Unbundle By Name(w110) -> ("ADAM"=w157:T43)
  n8 = Unbundle By Name("HDF5_file_refs") -> ("DO"=w106:bool[])
  n9 = Unbundle By Name(w110) -> ("Tone"=w152:T32[])
  n10 = Unbundle By Name(w110) -> ("TE"=w161:T42)
  n11 = Index Array(array=w42) -> (element=w41:T37)  [unwired: 1 in]
  n12 = for {
    tunnel: w43 -> [w220] mode=indexing
    tunnel: w41 -> [w201]
    tunnel: [w198] -> w40 mode=indexing
    tunnel: [w193] -> w39 mode=indexing
    tunnel: [w194] -> w38 mode=indexing
    tunnel: [w195] -> w37 mode=indexing
    tunnel: [w196] -> w36 mode=indexing
    tunnel: [w197] -> w35 mode=indexing
    tunnel: [w180] -> w34 mode=indexing
    tunnel: [w175] -> w33 mode=indexing
    tunnel: [w174] -> w32 mode=indexing
    tunnel: [w173] -> w31 mode=indexing
    # "Using \"Rain Rate\" for comparison to disdrometer\nbecause Rain Fall has 15-minute persistence.\nPer Nick. Luke 1-5-2022"
    n13 = Unbundle By Name(w201) -> ("DisdromSummary.Total Rain Rate"=w200:dbl, "DisdromSummary.Total Rain Rate"=w177:dbl, "DisdromSummary.Max Diameter Hail"=w186:dbl, "DisdromSummary.Total Rain Rate"=w184:dbl)
    n14 = Unbundle By Name(w220) -> ("Temperature"=w219:sgl, "Pressure"=w213:sgl, "Humidity"=w210:sgl, "Wind Speed"=w208:sgl, "Wind Dir"=w204:sgl, "Rain Fall"=w172:sgl, "Rain Rate"=w171:i16)
    n15 = Greater?(x=w200, y=12.0) -> (0:w183:bool)
    n16 = Greater?(x=w186, y=1.0) -> (0:w174:bool)
    n17 = Greater?(x=w184, y=250.0) -> (0:w173:bool)
    n18 = Equal To 0?(x=w171) -> (x = 0?=w182:bool)
    n19 = Equal To 0?(x=w177) -> (x = 0?=w179:bool)
    n20 = In Range and Coerce(upper limit=sgl 44.0, x=w219, lower limit=sgl -33.0) -> (In Range?=w216:bool)  [unwired: 1 out]
    n21 = In Range and Coerce(upper limit=sgl 1055.0, x=w213, lower limit=sgl 500.0) -> (In Range?=w192:bool)  [unwired: 1 out]
    n22 = In Range and Coerce(upper limit=sgl 100.0, x=w210, lower limit=sgl 0.0) -> (In Range?=w191:bool)  [unwired: 1 out]
    n23 = In Range and Coerce(upper limit=sgl 33.0, x=w208, lower limit=sgl 0.0) -> (In Range?=w190:bool)  [unwired: 1 out]
    n24 = In Range and Coerce(upper limit=sgl 360.0, x=w204, lower limit=sgl 0.0) -> (In Range?=w189:bool)  [unwired: 1 out]
    n25 = In Range and Coerce(upper limit=sgl 200.0, x=w172, lower limit=sgl 0.0) -> (In Range?=w188:bool)  [unwired: 1 out]
    n26 = Greater Than 0?(x=w171) -> (x > 0?=w178:bool)
    n27 = Select(t=w182, s=w183, f=FALSE) -> (s? t:f=w180:bool)
    n28 = Select(t=w179, s=w178, f=FALSE) -> (s? t:f=w175:bool)
    n29 = Not(x=w216) -> (.not. x?=w198:bool)
    n30 = Not(x=w192) -> (.not. x?=w193:bool)
    n31 = Not(x=w191) -> (.not. x?=w194:bool)
    n32 = Not(x=w190) -> (.not. x?=w195:bool)
    n33 = Not(x=w189) -> (.not. x?=w196:bool)
    n34 = Not(x=w188) -> (.not. x?=w197:bool)
  }
  n35 = Unbundle By Name("HDF5_file_refs") -> ("LogData.Tone"=w87:T32[])
  n36 = Index Array(array=w106, index #1=1 ("index"), index #2=2 ("index")) -> (element #1=w103:bool, element #2=w102:bool)
  n37 = Index Array(array=w101, index #1=0 ("index"), index #2=2 ("index")) -> (element #1=w98:T32, element #2=w97:T32)
  n38 = Unbundle By Name(w151) -> ("AI1"=w133:T46, "AI2"=w132:T46, "AI3"=w131:T46, "AI4"=w130:T46, "AI5"=w129:T46, "AI6"=w128:T46, "AI18"=w127:T46, "AI19"=w126:T46)  [unwired: 2 out]
  n39 = Unbundle By Name(w151) -> ("ADAM1"=w120:T46, "ADAM2"=w119:T46, "ADAM3"=w118:T46, "ADAM4"=w117:T46)
  n40 = Unbundle By Name(w157) -> ("Value 1"=w156:dbl, "Value 2"=w155:dbl, "Value 4"=w154:dbl, "Value 3"=w153:dbl)
  n41 = Unbundle By Name(w161) -> ("Temp"=w160:dbl, "Temp 2"=w159:dbl, "Temp 3"=w158:dbl)
  n42 = Unbundle By Name(w151) -> ("TC13"=w124:T46)
  n43 = Unbundle By Name(w151) -> ("TE1"=w123:T46, "TE2"=w122:T46, "TE3"=w121:T46)
  n44 = Unbundle By Name(w170) -> ("AI1_-5V"=w167:dbl, "AI2_+5V"=w166:dbl, "AI3_+6V"=w165:dbl, "AI4_+12V"=w164:dbl, "AI5_+15V"=w163:dbl, "AI6_+28V"=w162:dbl, "Ai18_InclinAz"=w116:dbl, "Ai19_InclinEl"=w115:dbl)  [unwired: 2 out]
  n45 = for {
    tunnel: w152 -> [w249] mode=indexing
    tunnel: w151 -> [w226]
    tunnel: [w234] -> w114 mode=indexing
    tunnel: [w232] -> w112 mode=indexing
    tunnel: [w236] -> w108 mode=indexing
    tunnel: [w227] -> w109 mode=indexing
    tunnel: w103 -> [w225]
    tunnel: w102 -> [w224]
    w244 = 1000000.0 ("Peak")
    n46 = Unbundle By Name(w249) -> ("BeacLoc"=w242:i32[], "CalLoc"=w243:i32[], "CalVal"=w230:sgl[])
    n47 = Unbundle By Name(w249) -> ("Enum"=w250:T15)
    n48 = case shown="\"4\"" w250 {
      tunnel: w226 -> [w274 w282 w295 w304]
      tunnel: [w271 w281 w288 w302] -> w248
      tunnel: [w268 w281 w289 w302] -> w247
      tunnel: [1 ("index") 2 ("index") 3 ("index") 4 ("index")] -> w237
      tunnel: [w267 w279 w290 w300] -> w231
      tunnel: w225 -> [w266 w278 _ _]
      tunnel: w224 -> [_ _ w287 w299]
      tunnel: ["72Co_BeacFreq" ("Source") "Nul" ("Source") "84Co_BeacFreq" ("Source") "Nul" ("Source")] -> w223
      tunnel: ["72Co_CalFreq" ("Source") "Nul" ("Source") "84Co_CalFreq" ("Source") "Nul" ("Source")] -> w222
      tunnel: ["72Co_CalPwr" ("Source") "72X_CalPwr" ("Source") "84Co_CalPwr" ("Source") "84X_CalPwr" ("Source")] -> w221
      frame "1" {
        n49 = Unbundle By Name(w274) -> ("72CoBeacFreq"=w272:T46, "72CoCalFreq"=w269:T46, "72Co_CalTonePwr"=w270:T46)
        n50 = call "EnableAlarm.vi"("Cal_Enable"=w266, "AlarmThresholds"=w272) -> ("AlarmThresholds out"=w271:T46)  [unwired: 9 in]
        n51 = call "EnableAlarm.vi"("Cal_Enable"=w266, "AlarmThresholds"=w269) -> ("AlarmThresholds out"=w268:T46)  [unwired: 9 in]
        n52 = call "EnableAlarm.vi"("Cal_Enable"=w266, "AlarmThresholds"=w270) -> ("AlarmThresholds out"=w267:T46)  [unwired: 9 in]
      }
      frame "2" {
        w281 = T46 {"Enbl"=FALSE, "ErrsAndWarns"={0.0, 0.0, 0.0, 0.0}} ("CalFreq")
        n53 = Unbundle By Name(w282) -> ("72X_CalTonePwr"=w280:T46)
        n54 = call "EnableAlarm.vi"("Cal_Enable"=w278, "AlarmThresholds"=w280) -> ("AlarmThresholds out"=w279:T46)  [unwired: 9 in]
      }
      frame "3" {
        n55 = Unbundle By Name(w295) -> ("84CoBeacFreq"=w293:T46, "84CoCalFreq"=w292:T46, "84Co_CalTonePwr"=w291:T46)
        n56 = call "EnableAlarm.vi"("Cal_Enable"=w287, "AlarmThresholds"=w293) -> ("AlarmThresholds out"=w288:T46)  [unwired: 9 in]
        n57 = call "EnableAlarm.vi"("Cal_Enable"=w287, "AlarmThresholds"=w292) -> ("AlarmThresholds out"=w289:T46)  [unwired: 9 in]
        n58 = call "EnableAlarm.vi"("Cal_Enable"=w287, "AlarmThresholds"=w291) -> ("AlarmThresholds out"=w290:T46)  [unwired: 9 in]
      }
      frame "4" {
        w302 = T46 {"Enbl"=FALSE, "ErrsAndWarns"={0.0, 0.0, 0.0, 0.0}} ("CalFreq")
        n59 = Unbundle By Name(w304) -> ("84X_CalTonePwr"=w301:T46)
        n60 = call "EnableAlarm.vi"("Cal_Enable"=w299, "AlarmThresholds"=w301) -> ("AlarmThresholds out"=w300:T46)  [unwired: 9 in]
      }
    }
    n61 = To Double Precision Float(number=w243) -> (double precision float=w240:dbl[])
    n62 = To Double Precision Float(number=w242) -> (double precision float=w241:dbl[])
    n63 = To Double Precision Float(number=w230) -> (double precision float=w229:dbl[])
    n64 = Divide(x=w241, y=w244) -> (x/y=w238:dbl[])
    n65 = Divide(x=w240, y=w244) -> (x/y=w239:dbl[])
    n66 = Absolute Value(x=w239) -> (abs(x)=w245:dbl[])
    n67 = Absolute Value(x=w238) -> (abs(x)=w246:dbl[])
    n68 = for {
      tunnel: w245 -> [w262] mode=indexing
      tunnel: w246 -> [w261] mode=indexing
      tunnel: w248 -> [w260]
      tunnel: w247 -> [w259]
      tunnel: [w258] -> w235 mode=indexing
      tunnel: [w257] -> w233 mode=indexing
      tunnel: w231 -> [w255]
      tunnel: w229 -> [w256] mode=indexing
      tunnel: [w254] -> w228 mode=indexing
      tunnel: w223 -> [w253]
      tunnel: w222 -> [w252]
      tunnel: w221 -> [w251]
      n69 = call "LimitTest.vi"("AlarmCfg"=w260, "Source"=w253, "Data"=w261) -> ("ErrorStatus"=w258:T2)  [unwired: 8 in]
      n70 = call "LimitTest.vi"("AlarmCfg"=w259, "Source"=w252, "Data"=w262) -> ("ErrorStatus"=w257:T2)  [unwired: 8 in]
      n71 = call "LimitTest.vi"("AlarmCfg"=w255, "Source"=w251, "Data"=w256) -> ("ErrorStatus"=w254:T2)  [unwired: 8 in]
    }
    n72 = call "OR_FreqErrors.vi"("Array"=w235) -> ("ErrorStatus"=w234:T2)  [unwired: 10 in]
    n73 = call "OR_FreqErrors.vi"("Array"=w233) -> ("ErrorStatus"=w232:T2)  [unwired: 10 in]
    n74 = call "OR_FreqErrors.vi"("Array"=w228) -> ("ErrorStatus"=w227:T2)  [unwired: 10 in]
    n75 = Decrement(x=w237) -> (x-1=w236:i32)
  }
  n76 = Unbundle By Name(w168) -> ("TC13_Amb_Inter"=w169:dbl)
  n77 = Unbundle By Name(w98) -> ("AboveThresh"=w55:bool[])
  n78 = Unbundle By Name(w97) -> ("AboveThresh"=w54:bool[])
  n79 = for {
    tunnel: w87 -> [w316] mode=indexing
    tunnel: [w311] -> w86 mode=indexing if=w314
    tunnel: [w310] -> w85 mode=indexing if=w314
    tunnel: [w309] -> w84 mode=indexing if=w314
    tunnel: [w308] -> w83 mode=indexing if=w314
    tunnel: [w307] -> w82 mode=indexing if=w314
    tunnel: [w306] -> w81 mode=indexing if=w314
    tunnel: [w311] -> w72 mode=indexing if=w305
    tunnel: [w310] -> w71 mode=indexing if=w305
    tunnel: [w309] -> w70 mode=indexing if=w305
    tunnel: [w308] -> w69 mode=indexing if=w305
    tunnel: [w307] -> w68 mode=indexing if=w305
    tunnel: [w306] -> w67 mode=indexing if=w305
    n80 = Unbundle By Name(w316) -> ("Enum"=w312:T15, "Saturat.Meas"=w311:bool[], "Saturat.Stage1"=w310:bool[], "Saturat.Stage4"=w309:bool[], "Saturat.Stage5"=w308:bool[], "Saturat.Stage6"=w307:bool[], "Saturat.Stage7"=w306:bool[])
    n81 = Equal?(x=TargetNumber."3", y=w312) -> (x = y?=w314:bool)
    n82 = Equal?(x=w312, y=TargetNumber."1" ("x")) -> (x = y?=w305:bool)
  }
  n83 = Empty Array?(array=w55) -> (empty?=w50:bool)
  n84 = Empty Array?(array=w54) -> (empty?=w52:bool)
  n85 = Or Array Elements(Boolean array=w55) -> (logical OR=w93:bool)
  n86 = Or Array Elements(Boolean array=w54) -> (logical OR=w92:bool)
  n87 = call "LimitTest.vi"("AlarmCfg"=w123, "Source"="TE1", "Data"=w160) -> ("ErrorStatus"=w141:T2)  [unwired: 8 in]
  n88 = call "LimitTest.vi"("AlarmCfg"=w120, "Source"="ADAM1", "Data"=w156) -> ("ErrorStatus"=w138:T2)  [unwired: 8 in]
  n89 = Or(x=w50, y=w93) -> (x .or. y?=w51:bool)
  n90 = call "LimitTest.vi"("AlarmCfg"=w122, "Source"="TE2", "Data"=w159) -> ("ErrorStatus"=w140:T2)  [unwired: 8 in]
  n91 = call "LimitTest.vi"("AlarmCfg"=w119, "Source"="ADAM2", "Data"=w155) -> ("ErrorStatus"=w137:T2)  [unwired: 8 in]
  n92 = Or(x=w92, y=w52) -> (x .or. y?=w53:bool)
  n93 = call "LimitTest.vi"("AlarmCfg"=w133, "Source"="AI1", "Data"=w167) -> ("ErrorStatus"=w149:T2)  [unwired: 8 in]
  n94 = call "LimitTest.vi"("AlarmCfg"=w121, "Source"="TE3", "Data"=w158) -> ("ErrorStatus"=w139:T2)  [unwired: 8 in]
  n95 = call "LimitTest.vi"("AlarmCfg"=w118, "Source"="ADAM3", "Data"=w154) -> ("ErrorStatus"=w136:T2)  [unwired: 8 in]
  n96 = call "LimitTest.vi"("AlarmCfg"=w132, "Source"="AI2", "Data"=w166) -> ("ErrorStatus"=w148:T2)  [unwired: 8 in]
  n97 = call "LimitTest.vi"("AlarmCfg"=w117, "Source"="ADAM4", "Data"=w153) -> ("ErrorStatus"=w135:T2)  [unwired: 8 in]
  n98 = call "LimitTest.vi"("AlarmCfg"=w131, "Source"="AI3", "Data"=w165) -> ("ErrorStatus"=w147:T2)  [unwired: 8 in]
  n99 = call "LimitTest.vi"("RX?"=w125, "AlarmCfg"=w124, "Source"="TC13", "Data"=w169) -> ("ErrorStatus"=w150:T2)  [unwired: 7 in]
  n100 = call "Elapsed Time"("Time Target (s)"=w94, "Reset"=w51) -> ("Elapsed Time (s)"=w91:dbl, "Time has Elapsed"=w48:bool)  [unwired: 10 in, 6 out]
  n101 = call "Elapsed Time2"("Time Target (s)"=w94, "Reset"=w53) -> ("Elapsed Time (s)"=w90:dbl, "Time has Elapsed"=w47:bool)  [unwired: 10 in, 6 out]
  n102 = call "LimitTest.vi"("AlarmCfg"=w130, "Source"="AI4", "Data"=w164) -> ("ErrorStatus"=w146:T2)  [unwired: 8 in]
  n103 = call "LimitTest.vi"("AlarmCfg"=w129, "Source"="AI5", "Data"=w163) -> ("ErrorStatus"=w145:T2)  [unwired: 8 in]
  n104 = call "LimitTest.vi"("AlarmCfg"=w128, "Source"="AI16", "Data"=w162) -> ("ErrorStatus"=w144:T2)  [unwired: 8 in]
  n105 = call "LimitTest.vi"("AlarmCfg"=w127, "Source"="AI18", "Data"=w116) -> ("ErrorStatus"=w143:T2)  [unwired: 8 in]
  n106 = Max & Min(x=w91, y=w90) -> (max(x,y)=→"Elapsed_SNR_Timer":dbl)  [unwired: 1 out]
  n107 = call "LimitTest.vi"("AlarmCfg"=w126, "Source"="AI19", "Data"=w115) -> ("ErrorStatus"=w142:T2)  [unwired: 8 in]
  n108 = Bundle By Name(cluster=T2 {"RX?"=FALSE, "Warn"=FALSE, "Error"=FALSE, "Enabl"=FALSE, "Source"=""}, "RX?"=TRUE, "Error"=w48, "Source"="72_SNR") -> (w95:T2)
  n109 = Or Array Elements(Boolean array=w86) -> (logical OR=w80:bool)
  n110 = Or Array Elements(Boolean array=w85) -> (logical OR=w79:bool)
  n111 = Or Array Elements(Boolean array=w84) -> (logical OR=w78:bool)
  n112 = Or Array Elements(Boolean array=w83) -> (logical OR=w77:bool)
  n113 = Or Array Elements(Boolean array=w82) -> (logical OR=w76:bool)
  n114 = Or Array Elements(Boolean array=w81) -> (logical OR=w75:bool)
  n115 = Or Array Elements(Boolean array=w72) -> (logical OR=w65:bool)
  n116 = Or Array Elements(Boolean array=w71) -> (logical OR=w64:bool)
  n117 = Or Array Elements(Boolean array=w70) -> (logical OR=w63:bool)
  n118 = Or Array Elements(Boolean array=w69) -> (logical OR=w62:bool)
  n119 = Or Array Elements(Boolean array=w68) -> (logical OR=w61:bool)
  n120 = Or Array Elements(Boolean array=w67) -> (logical OR=w60:bool)
  n121 = Or Array Elements(Boolean array=w40) -> (logical OR=w30:bool)
  n122 = Or Array Elements(Boolean array=w39) -> (logical OR=w29:bool)
  n123 = Or Array Elements(Boolean array=w38) -> (logical OR=w28:bool)
  n124 = Or Array Elements(Boolean array=w37) -> (logical OR=w27:bool)
  n125 = Or Array Elements(Boolean array=w36) -> (logical OR=w26:bool)
  n126 = Or Array Elements(Boolean array=w35) -> (logical OR=w25:bool)
  n127 = Or Array Elements(Boolean array=w34) -> (logical OR=w24:bool)
  n128 = Or Array Elements(Boolean array=w33) -> (logical OR=w23:bool)
  n129 = Or Array Elements(Boolean array=w32) -> (logical OR=w22:bool)
  n130 = Or Array Elements(Boolean array=w31) -> (logical OR=w21:bool)
  n131 = Build Array(w80, w79, w78, w77, w76, w75, w74, w74) -> (w58:bool[])
  n132 = Build Array(w65, w64, w63, w62, w61, w60, w66, w66) -> (w57:bool[])
  n133 = call "Sort_Tone_Errors.vi"("Array 3"=w114, "Array in"=w108) -> ("Array out"=w113:T2[])  [unwired: 9 in]
  n134 = call "Sort_Tone_Errors.vi"("Array 3"=w112, "Array in"=w108) -> ("Array out"=w111:T2[])  [unwired: 9 in]
  n135 = call "Sort_Tone_Errors.vi"("Array 3"=w109, "Array in"=w108) -> ("Array out"=w107:T2[])  [unwired: 9 in]
  n136 = Bundle By Name(cluster=T2 {"RX?"=FALSE, "Warn"=FALSE, "Error"=FALSE, "Enabl"=FALSE, "Source"=""}, "RX?"=TRUE, "Error"=w47, "Source"="84_SNR") -> (w45:T2)
  n137 = Build Array (concatenate)(w150, w149, w148, w147, w146, w145, w144, w143, w142, w141, w140, w139, w138, w137, w136, w135, w113, w111, w107, w95, w45) -> (w88:T2[])
  "AllAlarms" <- w88
  n138 = Build Array(w30, w29, w28, w27, w26, w25, w24, w23, w22, w21, w20, w20, w20, w20, w20, w20) -> (→"WeatherStatus":bool[])
  n139 = call "Sum_Erros.vi"("array error status"=w88) -> ("Alarms"=→"Alarm Status":T3)  [unwired: 10 in]
  n140 = Bundle By Name(cluster=T1 {"84"=[], "72"=[]}, "84"=w58, "72"=w57) -> (→"SaturationStatus":T1)
